vi "utilities_setProperties.vi"(6 "sheet name":string, 8 "error in (no error)":errorcluster, 9 "title":string, 10 "creator":string, 11 "Excel refnum":T1) -> (0 "error out":errorcluster, 3 "Excel refnum out":T1)   [LabVIEW 2017, in "NI_ExcelFile.lvlib"]
uses:
  <vilib>/express/express shared/NI_ExcelFile/NI_ExcelFile.lvlib
  <vilib>/express/express shared/NI_ExcelFile/Ctrls/ExcelRefnum.ctl
  <vilib>/express/express shared/NI_ExcelFile/Ctrls/MainData.ctl
  <vilib>/express/express shared/NI_ExcelFile/Ctrls/StreamMode.ctl
  <vilib>/express/express shared/NI_ExcelFile/Ctrls/TimeColumnMode.ctl
  <vilib>/express/express shared/NI_ExcelFile/Ctrls/FileAttribute.ctl
  <vilib>/express/express shared/NI_ExcelFile/Ctrls/Columns.ctl
  <vilib>/express/express shared/NI_ExcelFile/Ctrls/ColumnInfo.ctl
  <vilib>/express/express shared/NI_ExcelFile/Ctrls/DataType.ctl
  <vilib>/express/express shared/NI_ExcelFile/Ctrls/wd_recordInfo.ctl
  <vilib>/express/express shared/NI_ExcelFile/Ctrls/disk_TemplateFile.ctl
  <vilib>/express/express shared/NI_ExcelFile/Ctrls/meta_file.ctl
  <vilib>/express/express shared/NI_ExcelFile/Ctrls/meta_Block.ctl
  <vilib>/express/express shared/NI_ExcelFile/Ctrls/meta_BlockType.ctl
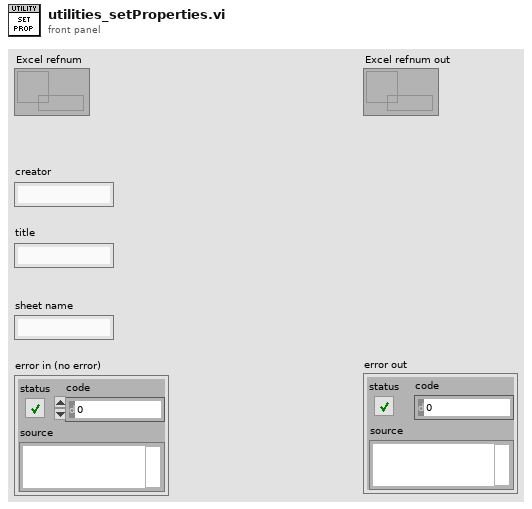
[diagram p1: front panel]
types:
  T1 = typedef "NI_ExcelFile.lvlib/ExcelRefnum.ctl" = refnum<data-value>
  T2 = typedef "NI_ExcelFile.lvlib/MainData.ctl" = cluster{"TargetFile":path, "StreamMode":T3, "Append?":bool, "ChunkSize":u64, "TimeColumnMode":T4, "TimestampFormat":string, "AbsoluteTime?":bool, "FileAttribute ":T5, "Column":T6, "FileRef":refnum<k1>, "MemoryRef":refnum<data-value>[], "RecordInfo":T9[], " ChannelPreviousInfo":u32[], "ChannelFirstRecord":u32[], "PredefinedFormattedValueLength":i64, "DiskTemplate":T10}
  T3 = typedef "NI_ExcelFile.lvlib/StreamMode.ctl" = enum16{"File", "Memory"}
  T4 = typedef "NI_ExcelFile.lvlib/TimeColumnMode.ctl" = enum16{"Empty", "OnePerCh", "One"}
  T5 = typedef "NI_ExcelFile.lvlib/FileAttribute.ctl" = cluster{"Creator":string, "Title":string, "SheetName":string}
  T6 = typedef "NI_ExcelFile.lvlib/Columns.ctl" = T7[]
  T7 = typedef "NI_ExcelFile.lvlib/ColumnInfo.ctl" = cluster{"Header":string, "Format":string, "DataType":T8, "Length":u64}
  T8 = typedef "NI_ExcelFile.lvlib/DataType.ctl" = enum16{"DDT", "WFM", "Array of STR", "Array of DBL", "Array of I8", "Array of I16", "Array of I32", "Array of I64", "Array of SGL", "Array of U8", "Array of U16", "Array of U32", "Array of U64", "Array of Time"}
  T9 = typedef "NI_ExcelFile.lvlib/wd_recordInfo.ctl" = cluster{"ChannelIndex":u32, "StartIndex":u64, "Length":u64, "Previous":i32, "Next":i32}
  T10 = typedef "NI_ExcelFile.lvlib/disk_TemplateFile.ctl" = cluster{"XMLRef":refnum<file>[], "ZipPath":path, "MetaFile":T11, "TempFolder":path}
  T11 = typedef "NI_ExcelFile.lvlib/meta_file.ctl" = cluster{"Ref":refnum<file>, "NextRow":i32, "NextPosition":i64, "Block":T12[]}
  T12 = typedef "NI_ExcelFile.lvlib/meta_Block.ctl" = cluster{"Version":u16, "Type":T13, "Length":i32, "Data":string}
  T13 = typedef "NI_ExcelFile.lvlib/meta_BlockType.ctl" = enum16{"NITag", "File", "Column"}
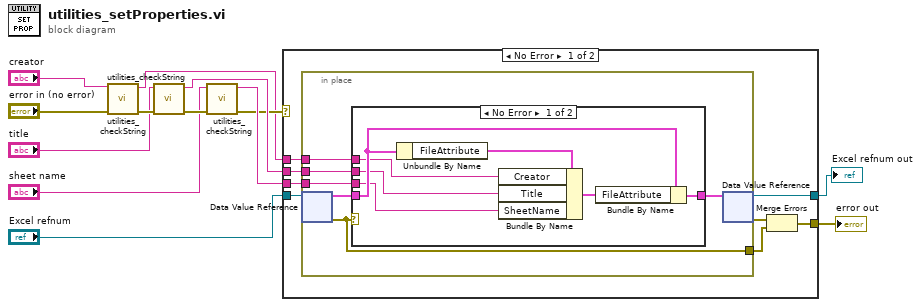
[diagram p0: block diagram]
diagram:
  n1 = call <vilib>:"utilities_checkString.vi"("error in (no error)"="error in (no error)", "String"="creator") -> ("error out"=w8:errorcluster, "String out"=w1:string)  [unwired: 8 in]
  n2 = call <vilib>:"utilities_checkString.vi"("error in (no error)"=w8, "String"="title") -> ("error out"=w6:errorcluster, "String out"=w5:string)  [unwired: 8 in]
  n3 = call <vilib>:"utilities_checkString.vi"("error in (no error)"=w6, "String"="sheet name") -> ("error out"=w2:errorcluster, "String out"=w3:string)  [unwired: 8 in]
  n4 = case shown="No Error" w2 {
    selector: w2 -> [_ w36]
    tunnel: "Excel refnum" -> [w21 w37]
    tunnel: w1 -> [w20 _]
    tunnel: w5 -> [w19 _]
    tunnel: w3 -> [w18 _]
    tunnel: [w17 w37] -> w12
    tunnel: [w14 w36] -> w11
    frame No Error {
      n5 = in-place {
        in-place-border: w20 -> [w26]
        in-place-border: w19 -> [w25]
        in-place-border: w18 -> [w24]
        in-place-border: [w22] -> w15
        n6 = in-place-dvr #1(w21) -> (w27:T2, w22:errorcluster)
        n7 = case shown="No Error" w22 {
          tunnel: w27 -> [w34 w35]
          tunnel: w26 -> [w32 _]
          tunnel: w25 -> [w31 _]
          tunnel: w24 -> [w30 _]
          tunnel: [w28 w35] -> w23
          frame No Error {
            n8 = Unbundle By Name(w34) -> ("FileAttribute"=w33:T5)
            n9 = Bundle By Name(cluster=w33, "Creator"=w32, "Title"=w31, "SheetName"=w30) -> (w29:T5)
            n10 = Bundle By Name(cluster=w34, "FileAttribute"=w29) -> (w28:T2)
          }
          frame Error {
          }
        }
        n11 = in-place-dvr #1(w23) -> (w17:T1, w16:errorcluster)
      }
      n12 = Merge Errors(w16, w15) -> (w14:errorcluster)
    }
    frame Error {
    }
  }
  "Excel refnum out" <- w12
  "error out" <- w11
